vi "GCSArray_load_file.vi"(0 "GCS Array Filepath":path, 5 "error in (no error)":errorcluster, 6 "Block index":i32 min=0 max=0) -> (14 "GCSArray data":dbl[][](array[numeric]), 19 "error out":errorcluster)   [LabVIEW 2026]
doc: "Load specified GCSArray from file into 2D double array."
uses:
  GCSArray_regex_selector.ctl
  GCSArray_regex_range.ctl
panel:
  # "Load specified GCSArray from file into 2D double array."
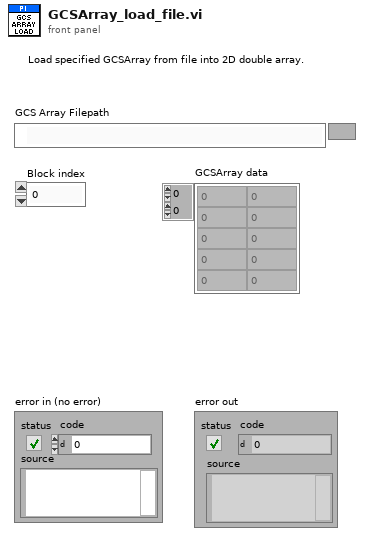
[diagram p1: front panel]
types:
  T1 = typedef "GCSArray_regex_range.ctl" = cluster{"Begin":i32, "End":i32}
  T2 = typedef "GCSArray_regex_selector.ctl" = enum16{"GCS_ARRAY Block Full", "GCS_ARRAY Block ID", "GCS_ARRAY Block Header", "GCS_ARRAY Block Data", "GCS_ARRAY Identifier", "GCS_ARRAY Remark", "GCS_ARRAY Version", "GCS_ARRAY Dimension", "GCS_ARRAY Type", "GCS_ARRAY Separator", "GCS_ARRAY NData", "GCS_ARRAY NData%", "GCS_ARRAY NData% Keyword", "GCS_ARRAY Name%", "GCS_ARRAY Name% Keyword", "GCS_ARRAY Start%", "GCS_ARRAY Start% Keyword", "GCS_ARRAY End%", "GCS_ARRAY End% Keyword", "GCS_ARRAY Delta%", "GCS_ARRAY Delta% Keword", "GCS_ARRAY Sample Time", "GCS_ARRAY Unit of transmitted value%", "GCS_ARRAY Trans_Unit% Keyword", "GCS_ARRAY Trans_Unit% = RAW Keyword", "GCS_ARRAY Unit of displayed value%", "GCS_ARRAY Disp_Unit% Keyword", "GCS_ARRAY Nominator%", "GCS_ARRAY Ratio_Nom% Keyword", "GCS_ARRAY Denominator%", "GCS_ARRAY Ratio_Denom% Keyword", "GCS_ARRAY End of Header", "GCS_ARRAY Empty line of Header"}
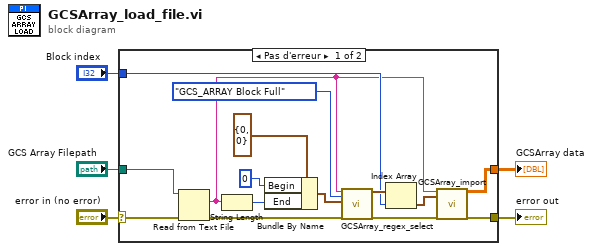
[diagram p0: block diagram]
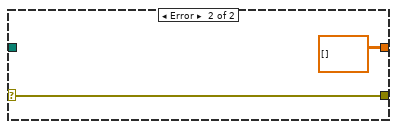
[diagram p2: hidden frame]
diagram:
  n1 = case shown="Pas d'erreur" "error in (no error)" {
    selector: "error in (no error)" -> [w19 w22]
    tunnel: [w18 w22] -> w4
    tunnel: [w17 dbl[][] [] ("GCSArray data")] -> w3
    tunnel: "Block index" -> [w10 _]
    tunnel: "GCS Array Filepath" -> [w20 _]
    frame No Error {
      n2 = Read from Text File(file (use dialog)=w20, error in=w19) -> (text=w7:string, error out=w13:errorcluster)  [unwired: 4 out]
      n3 = String Length(string=w7) -> (length=w14:i32)
      n4 = Bundle By Name(cluster=T1 {"Begin"=0, "End"=0} ("Selection"), "Begin"=0, "End"=w14) -> (w9:T1)
      n5 = call "GCSArray_regex_select.vi"("GCSArray input string"=w7, "Selector"=GCSArray_regex_selector."GCS_ARRAY Block Full", "Range"=w9, "error in (no error)"=w13) -> ("Matches"=w11:T1[], "error out"=w12:errorcluster)  [unwired: 14 out]
      n6 = Index Array(array=w11, index=w10) -> (element=w6:T1)
      n7 = call "GCSArray_import.vi"("GCSArray input string"=w7, "Range"=w6, "error in (no error)"=w12) -> ("GCSArray data"=w17:dbl[][], "error out"=w18:errorcluster)  [unwired: 15 out]
    }
    frame Error {
    }
  }
  "error out" <- w4
  "GCSArray data" <- w3
